vi "Globals HCC.vi"() -> ()   [LabVIEW 2012]
panel:
  in  "Resend Enable Log Period":u32=15
  in  "Error Count Limit":u32=60
  in  "Color Run":u32(colorbox)=6618880
  in  "Color Caution":u32(colorbox)=16776960
  in  "Sub Comma":string=" "
  in  "No Port MSG":string="Unconfigured Port"
  in  "Filename Suffix":string="Washer_Debug_Log.csv"
  in  "Sample Data Preamble Header":string[][](array[string])=[["computer", "", "Location->"], ["Index", "Date(Y-m-d)", "Time"]]
  in  "Max Length of Display Data":i32=10000
  in  "Label Com Array":string[][](array[string])=[["M1", "100"], ["M3", "3"], ["M5", "5"], ["M7", "7"], ["M9", "9"], ["M11", "11"], ["M13", "13"], ["M15", "15"], ["M17", "17"], ["M19", "19"], ["M2", "2"], ["M4", "4"], ["M6", "6"], ["M8", "8"], ["M10", "10"], ["M12", "12"], ["M14", "14"], ["M16", "16"], ["M18", "18"], ["M20", "20"], ["N6", "21"], ["N7", "22"], ["N8", "23"], ["N9", "24"], ["N10", "25"], ["N11", "26"], ["N12", "27"], ["N13", "28"]]
  in  "Sub /R/N":string=" :: "
  in  "Path: Data Backup":path=path "\\\\192.168.1.12\\share/Test Data/HCC"
  in  "Sample Header Data":string[](array[string])=["Debug Data"]
  in  "Color Uncofigured":u32(colorbox)=7171459
  in  "Color Configured":u32(colorbox)=16860
  in  "Color No Com":u32(colorbox)
  in  "No Com Status Message":string="No Com"
  in  "Path: Save File":path=path "C:/data"
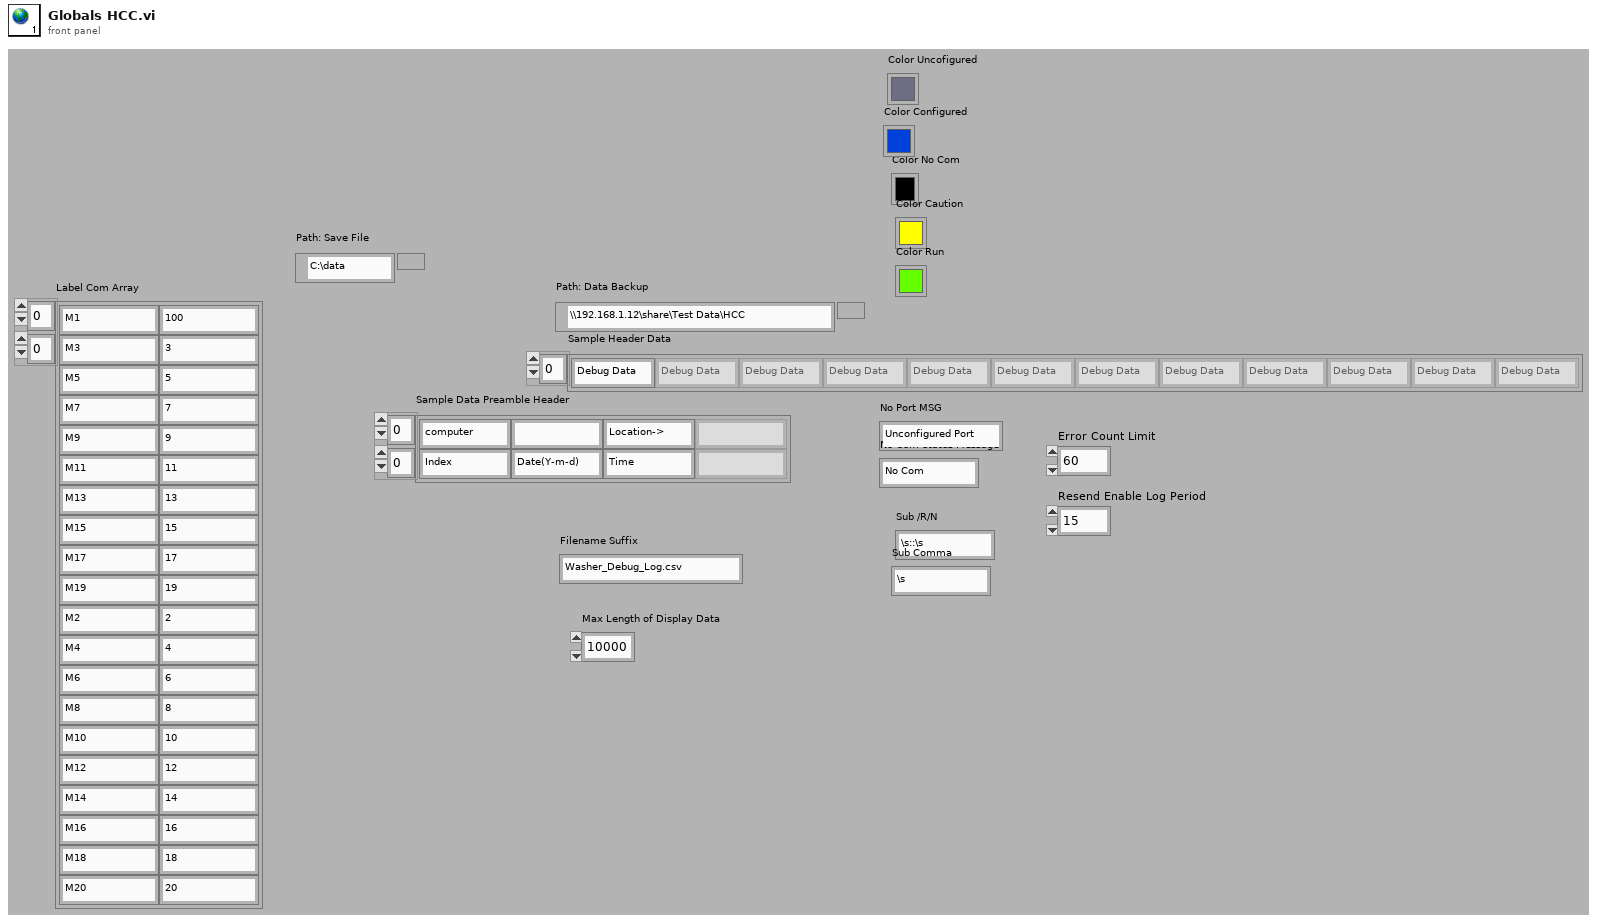
[diagram p1: front panel]
diagram:
